vi "Solve1.vi"(8 "Error In":errorcluster, 11 "object in":refnum<class "2021_21.lvclass">) -> (0 "Error Out":errorcluster, 2 "Result":u64, 3 "object out":refnum<class "2021_21.lvclass">)   [LabVIEW 2020, in "2021_21.lvclass"]
uses:
  2021_21.lvclass
  2021_21.lvclass/2021_21.ctl
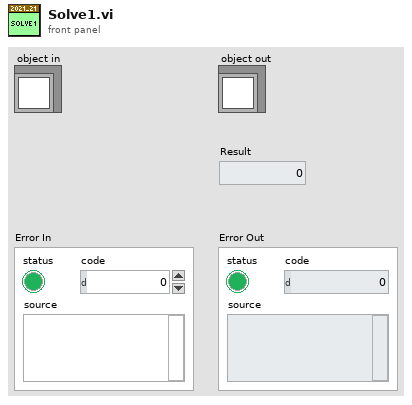
[diagram p1: front panel]
types:
  T1 = cluster{"DiceValue":i32, "P1_Pos":i32, "P2_Pos":i32, "P1_Score":i32, "P2_Score":i32, "DiceRolled":i32}
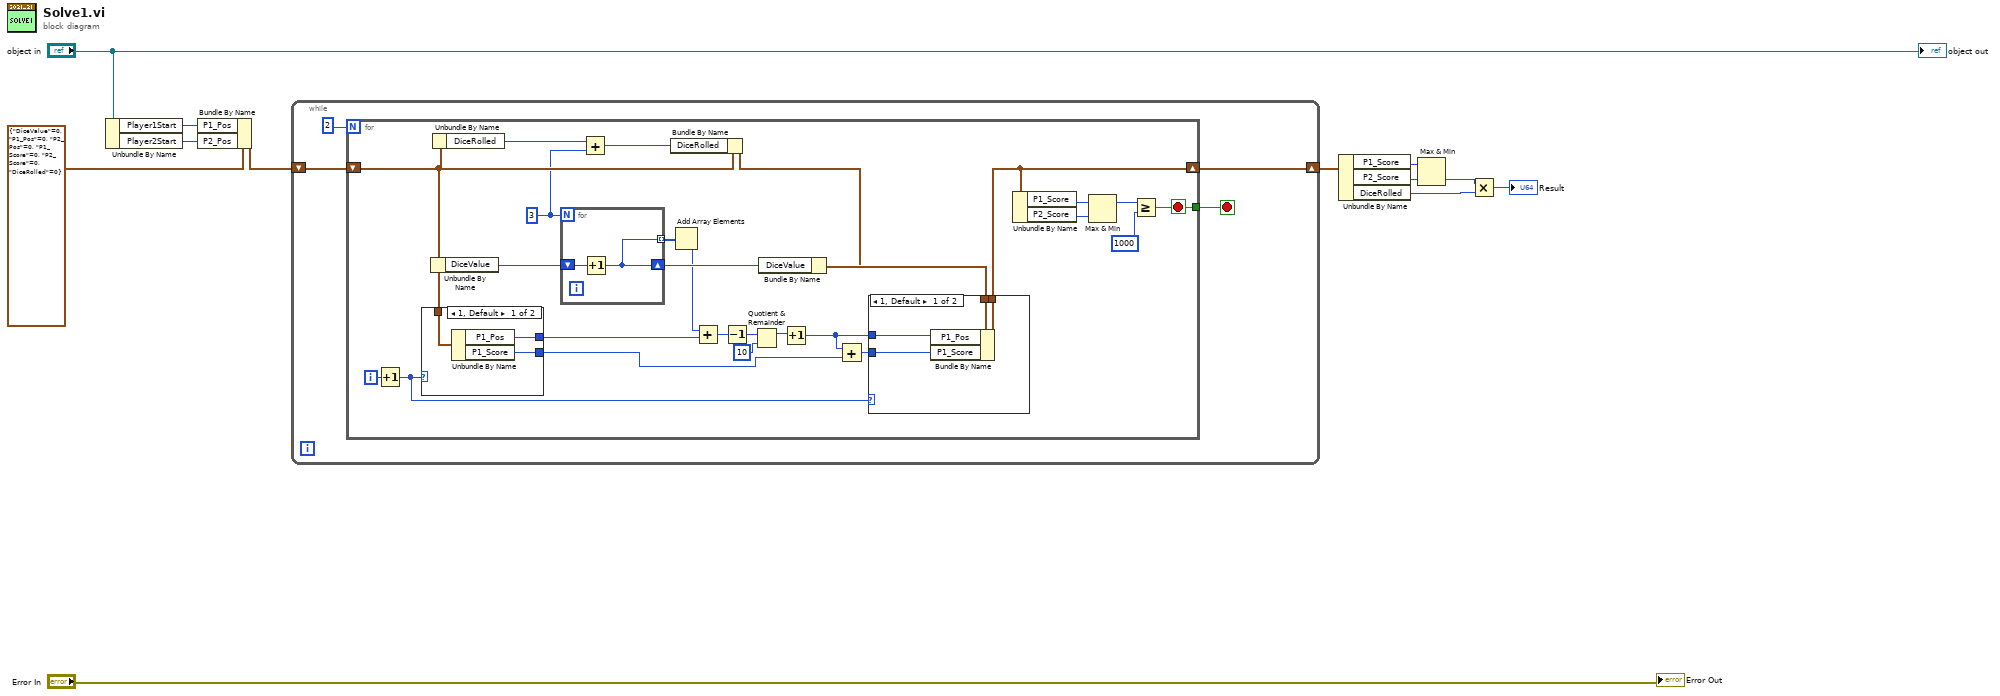
[diagram p0: block diagram]
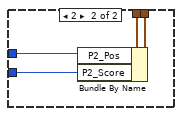
[diagram p2: hidden frame]
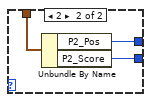
[diagram p3: hidden frame]
diagram:
  n1 = Unbundle By Name("object in") -> ("Player1Start"=w8:i32, "Player2Start"=w7:i32)
  n2 = Bundle By Name(cluster=T1 {"DiceValue"=0, "P1_Pos"=0, "P2_Pos"=0, "P1_Score"=0, "P2_Score"=0, "DiceRolled"=0}, "P1_Pos"=w8, "P2_Pos"=w7) -> (w10:T1)
  n3 = while {
    shift-right: [w13] -> w4
    shift-left: w10 -> [w16]
    stop <- w14 stop-if-true
    n4 = for {
      N: 2 -> [_]
      shift-right: [w31] -> w13
      shift-left: w16 -> [w20]
      tunnel: [w26] -> w14
      i -> [w33]
      stop <- w26 stop-if-true
      w18 = 3
      n5 = Increment(x=w33) -> (x+1=w25:i32)
      n6 = case shown="1, Default" w25 {
        tunnel: w20 -> [w53 w56]
        tunnel: [w52 w55] -> w38
        tunnel: [w51 w54] -> w23
        frame 1, Default {
          n7 = Unbundle By Name(w53) -> ("P1_Pos"=w52:i32, "P1_Score"=w51:i32)
        }
        frame 2 {
          n8 = Unbundle By Name(w56) -> ("P2_Pos"=w55:i32, "P2_Score"=w54:i32)
        }
      }
      n9 = Unbundle By Name(w20) -> ("DiceValue"=w41:i32)
      n10 = Unbundle By Name(w20) -> ("DiceRolled"=w19:i32)
      n11 = for {
        N: w18 -> [_]
        shift-right: [w57] -> w40
        shift-left: w41 -> [w58]
        tunnel: [w57] -> w42 mode=indexing
        n12 = Increment(x=w58) -> (x+1=w57:i32)
      }
      n13 = Add(x=w19, y=w18) -> (x+y=w17:i32)
      n14 = Bundle By Name(cluster=w20, "DiceRolled"=w17) -> (w21:T1)
      n15 = Add Array Elements(numeric array=w42) -> (sum=w39:i32)
      n16 = Add(x=w39, y=w38) -> (x+y=w37:i32)
      n17 = Decrement(x=w37) -> (x-1=w35:i32)
      n18 = Quotient & Remainder(x=w35, y=10) -> (x-y*floor(x/y)=w34:i32)  [unwired: 1 out]
      n19 = Bundle By Name(cluster=w21, "DiceValue"=w40) -> (w32:T1)
      n20 = Increment(x=w34) -> (x+1=w24:i32)
      n21 = Add(x=w24, y=w23) -> (x+y=w22:i32)
      n22 = case shown="1, Default" w25 {
        tunnel: w32 -> [w46 w50]
        tunnel: [w45 w49] -> w31
        tunnel: w24 -> [w44 w48]
        tunnel: w22 -> [w43 w47]
        frame 1, Default {
          n23 = Bundle By Name(cluster=w46, "P1_Pos"=w44, "P1_Score"=w43) -> (w45:T1)
        }
        frame 2 {
          n24 = Bundle By Name(cluster=w50, "P2_Pos"=w48, "P2_Score"=w47) -> (w49:T1)
        }
      }
      n25 = Unbundle By Name(w31) -> ("P1_Score"=w30:i32, "P2_Score"=w29:i32)
      n26 = Max & Min(x=w30, y=w29) -> (max(x,y)=w28:i32)  [unwired: 1 out]
      n27 = Greater Or Equal?(x=w28, y=1000) -> (x >= y?=w26:bool)
    }
  }
  n28 = Unbundle By Name(w4) -> ("P1_Score"=w5:i32, "P2_Score"=w6:i32, "DiceRolled"=w2:i32)
  n29 = Max & Min(x=w5, y=w6) -> (min(x,y)=w3:i32)  [unwired: 1 out]
  n30 = Multiply(x=w3, y=w2) -> (x*y=→"Result":i32)
  "Error Out" <- "Error In"
  "object out" <- "object in"
